vi "New_group_menu.vi"(0 "Enable":bool=TRUE, 5 "error in (no error)":errorcluster) -> (17 "Please Enter New Group":string, 18 "Add new group":bool, 19 "error out":errorcluster)   [LabVIEW 2012]
doc: "Displays a standard dialog box that prompts users to enter information, such as a user name and password.\n--------------------\n\nThis Express VI is configured as follows:\n\nMessage to Display to the User:Test\nThe inputs are: \nText Entry Box: Please Enter New Group"
panel:
  in  "New Experiment Group ID:":string="New Group Name" caption="Please Enter New Group"
  in  "OK2":bool
  in  "Cancel":bool
  in  "Please Select Group:":u16(ring) items=["CCLDAS"=1, "LASP"=2, "CU"=3, "Team Awesome"=4]
  in  "Please Enter an Experiment Description:":string caption="Please Enter Experiment Description:"
  in  "Please Enter an Experiment Name:":string caption="Please Enter Tags:"
  # "Please Enter New Experiment Group ID For Storage in the CCLDAS Database."
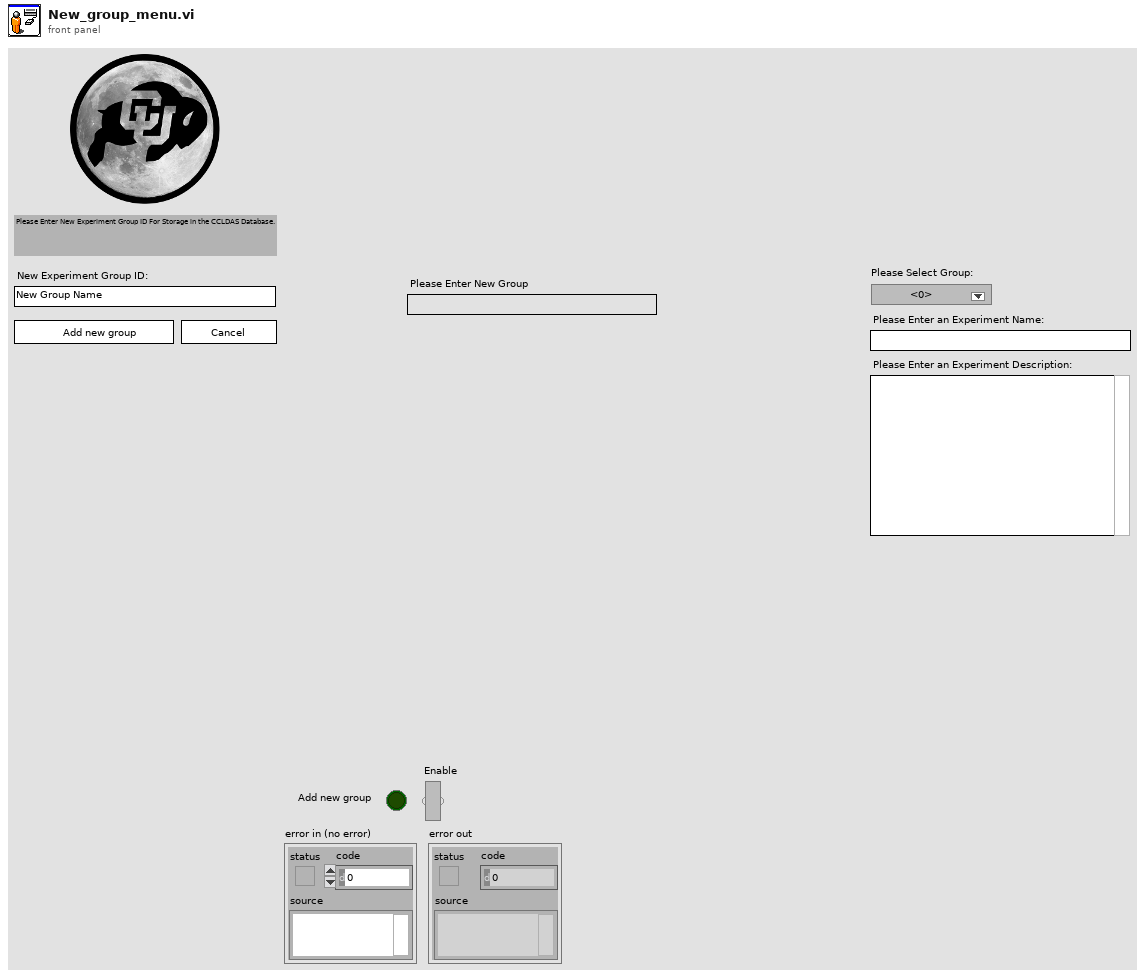
[diagram p1: front panel]
types:
  T1 = cluster{"Input Name":string, "Input Data Type":i32}[]
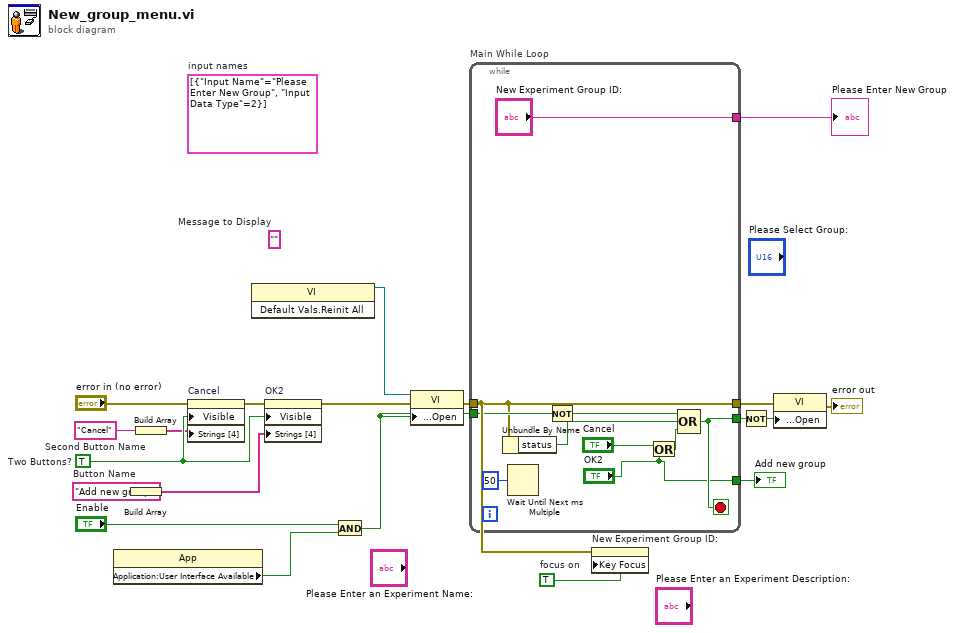
[diagram p0: block diagram]
diagram:
  w2 = TRUE  # focus on
  (unwired) T1 [{"Input Name"="Please Enter New Group", "Input Data Type"=2}]  # input names
  w14 = "Cancel"  # Second Button Name
  w12 = "Add new group"  # Button Name
  (unwired) ""  # Message to Display
  w20 = TRUE  # Two Buttons?
  n1 = property class="App"() -> ("Application:User Interface Available"=w5:bool)  [unwired: 2 in, 2 out]
  n2 = Build Array(w12) -> (w13:string[])
  n3 = Build Array(w14) -> (w15:string[])
  n4 = property on="Cancel" class="Bool"(error in="error in (no error)", "Visible"=w20, "Strings [4]"=w15) -> (error out=w18:errorcluster)  [unwired: 1 in, 1 out]
  n5 = invoke class="VI" method="Default Vals.Reinit All"() -> (reference out=w4:refnum<vi>)  [unwired: 3 in, 2 out]
  n6 = property on="OK2" class="Bool"(error in=w18, "Visible"=w20, "Strings [4]"=w13) -> (error out=w1:errorcluster)  [unwired: 1 in, 1 out]
  n7 = And(x="Enable", y=w5) -> (x .and. y?=w6:bool)
  n8 = property class="VI"(reference=w4, error in=w1, "Front Panel Window:Open"=w6) -> (error out=w11:errorcluster)  [unwired: 1 out]
  n9 = while "Main While Loop" {
    tunnel: ["OK2"] -> w19
    tunnel: w6 -> [w28]
    tunnel: [w26] -> w16
    tunnel: w11 -> [w25]
    tunnel: [w25] -> w9
    tunnel: ["New Experiment Group ID:"] -> w3
    stop <- w26 stop-if-true
    n10 = Unbundle By Name(w25) -> ("status"=w23:bool)
    n11 = Wait Until Next ms Multiple(millisecond multiple=u32 50) -> ()  [unwired: 1 out]
    n12 = Not(x=w28) -> (.not. x?=w27:bool)
    n13 = Or(x="Cancel", y="OK2") -> (x .or. y?=w24:bool)
    n14 = Compound Arithmetic op=OR(w27, w23, w24) -> (w26:bool)
  }
  "Add new group" <- w19
  "Please Enter New Group" <- w3
  n15 = property on="New Experiment Group ID:" class="Str"(error in=w11, "Key Focus"=w2) -> ()  [unwired: 1 in, 2 out]
  n16 = Not(x=w16) -> (.not. x?=w17:bool)
  n17 = property class="VI"(error in=w9, "Front Panel Window:Open"=w17) -> (error out=→"error out":errorcluster)  [unwired: 1 in, 1 out]
